vi "Dispatch Start.vi"(8 "error in (no error)":errorcluster, 11 "Dispatcher in":refnum<class "Dispatcher Thread.lvclass">) -> (0 "error out":errorcluster, 3 "Dispatcher out":refnum<class "Dispatcher Thread.lvclass">)   [LabVIEW 2017, in "DSF Core.lvlib" / "Dispatcher Thread.lvclass"]
uses:
  Dispatcher Thread.lvclass
  Interface/Dispatcher/Response Data.ctl
  Interface/Dispatcher/Response.ctl
  Interface/Dispatcher/Parameters.ctl
  Dispatcher Thread.lvclass/Dispatcher Thread.ctl
  Pool/Plugin Interface/Plugin Interface Pool.lvclass/Plugin Interface Pool.ctl
  Interface/Dispatcher/Write.vi
  Interface/Dispatcher/Write Dispatcher Response.vi
  Pool/Plugin Interface/Plugin Interface Pool.lvclass
  Interface/Dispatcher/Dispatcher Interface.lvclass
  Interface/Plugin/Plugin Interface.lvclass
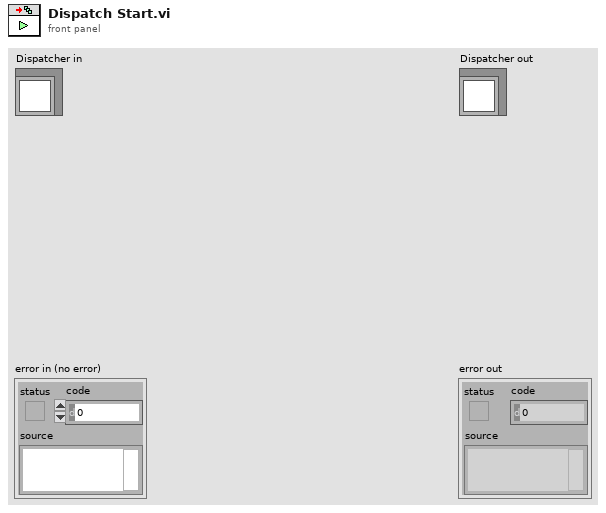
[diagram p1: front panel]
types:
  T1 = typedef "DSF Core.lvlib/Dispatcher Interface.lvclass/Response.ctl" = enum8{"General Ack", "Error", "Shutting Down"}
  T2 = typedef "DSF Core.lvlib/Dispatcher Interface.lvclass/Response Data.ctl" = cluster{"Response":T1, "Parameters":T3}
  T3 = typedef "DSF Core.lvlib/Dispatcher Interface.lvclass/Parameters.ctl" = cluster{"arg1":u64, "arg2":u64}
  T4 = typedef "DSF Core.lvlib/Dispatcher Thread.lvclass/Plugin Settings.ctl" = cluster{"Transfer Group threads":i32[], "Plugin Thread Pool":refnum<class "Plugin Interface Pool.lvclass">}
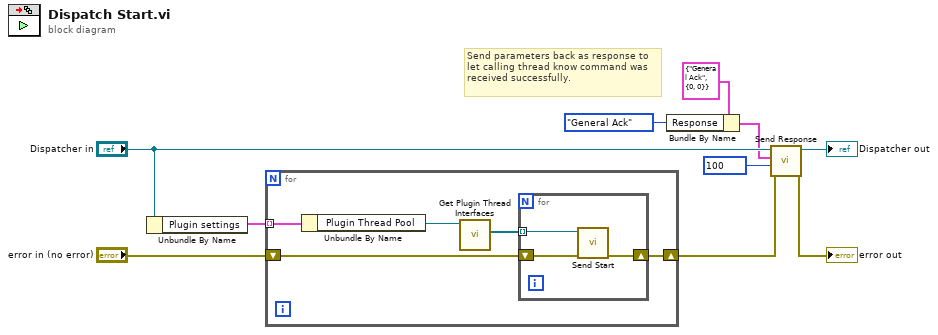
[diagram p0: block diagram]
diagram:
  # "Send parameters back as response to let calling thread know command was received successfully."
  n1 = Unbundle By Name("Dispatcher in") -> ("Plugin settings"=w10:T4[])
  n2 = for {
    tunnel: w10 -> [w12] mode=indexing
    shift-right: [w14] -> w7
    shift-left: "error in (no error)" -> [w13]
    n3 = Unbundle By Name(w12) -> ("Plugin Thread Pool"=w11:refnum<class "Plugin Interface Pool.lvclass">)
    n4 = call "Get Plugin Thread Interfaces.vi"("Plugin Interface Pool in"=w11) -> ("Plugin Thread Interfaces"=w15:refnum<class "Plugin Interface.lvclass">[])  [unwired: 9 in, 1 out]
    n5 = for {
      tunnel: w15 -> [w18] mode=indexing
      shift-right: [w16] -> w14
      shift-left: w13 -> [w17]
      n6 = call "Send Start.vi"("error in (no error)"=w17, "Plugin Interface in"=w18) -> ("error out"=w16:errorcluster)  [unwired: 8 in, 1 out]
    }
  }
  n7 = Bundle By Name(cluster=T2 {"Response"=enum."General Ack", "Parameters"={"arg1"=0, "arg2"=0}} ("response"), "Response"=Response."General Ack") -> (w1:T2)
  n8 = call "Send Response.vi"("error in (no error)"=w7, "timeout in ms (0)"=100, "response"=w1, "Dispatcher in"="Dispatcher in") -> ("error out"=→"error out":errorcluster, "Dispatcher out"=→"Dispatcher out":refnum<class "Dispatcher Thread.lvclass">)  [unwired: 6 in]
